vi "Intake_Notifier_Begin.vi"   [LabVIEW 2020]
uses:
  Intake_control_states.ctl
  Intake_cluster.ctl
  Globals/Intake_Globals.vi
types:
  T1 = typedef "Intake_cluster.ctl" = cluster{"control_states":T2, "%Vbus":dbl, "Trigger?":bool, "Manual_Extend?":bool, "Auto_Notifier":refnum<notifier>, "Step":dbl, "Parameter 1":dbl, "Parameter 2":dbl, "Parameter 3":dbl}
  T2 = typedef "Intake_control_states.ctl" = enum16{"No_Op", "Intake", "Manual", "Outtake"}
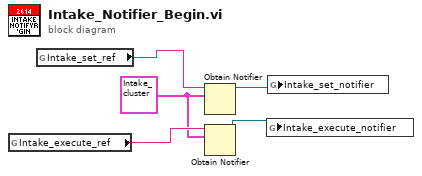
[diagram p0: block diagram]
diagram:
  w1 = T1 {"control_states"=enum."Intake", "%Vbus"=0.0, "Trigger?"=FALSE, "Manual_Extend?"=FALSE, "Auto_Notifier"=refnum, "Step"=0.0, "Parameter 1"=0.0, "Parameter 2"=0.0, "Parameter 3"=0.0}
  n1 = global read "Intake_Globals.vi" "Intake_execute_ref"() -> (w3:string)
  n2 = global read "Intake_Globals.vi" "Intake_set_ref"() -> (w2:string)
  n3 = Obtain Notifier(name (unnamed)=w2, notification data type=w1) -> (notifier out=w4:refnum<notifier>)  [unwired: 2 in, 2 out]
  n4 = Obtain Notifier(name (unnamed)=w3, notification data type=w1) -> (notifier out=w5:refnum<notifier>)  [unwired: 2 in, 2 out]
  n5 = global write "Intake_Globals.vi" "Intake_execute_notifier"(w5) -> ()
  n6 = global write "Intake_Globals.vi" "Intake_set_notifier"(w4) -> ()
